vi "dataset.update_set_property.vi"(8 "error in":errorcluster, 11 "DatasetUpdateStaging in":refnum<class "DatasetUpdateStaging.lvclass">) -> (0 "error out":errorcluster, 3 "DatasetUpdateStaging out":refnum<class "DatasetUpdateStaging.lvclass">)   [LabVIEW 2020, in "DatasetUpdateStaging.lvclass"]
doc: "Sets a property (key and value) on the dataset update being staged, replacing the dataset's entire property set on commit."
uses:
  DatasetUpdateStaging.lvclass
  DatasetUpdateStaging.lvclass/DatasetUpdateStaging.ctl
  client.lvlib
panel:
  in  "key":string
  in  "value":string
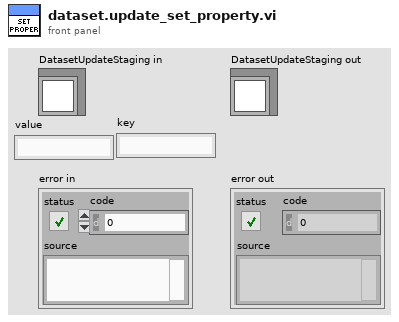
[diagram p1: front panel]
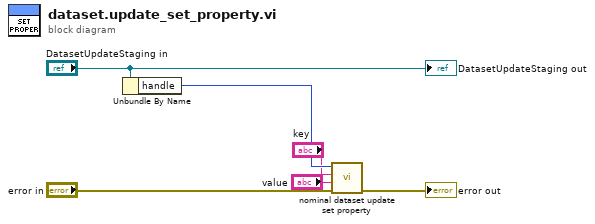
[diagram p0: block diagram]
diagram:
  n1 = Unbundle By Name("DatasetUpdateStaging in") -> ("handle"=w4:i32)
  n2 = call "nominal dataset update set property.vi"("error in (no error)"="error in", "value"="value", "key"="key", "staging"=w4) -> ("error out"=→"error out":errorcluster)  [unwired: 6 in, 1 out]
  "DatasetUpdateStaging out" <- "DatasetUpdateStaging in"
